vi "Create Request.vi"(8 "error in (no error)":errorcluster, 10 "request":T1, 11 "JSON-RPC in":refnum<class "JSON-RPC.lvclass">) -> (0 "error out":errorcluster, 2 "Request":string, 3 "JSON-RPC out":refnum<class "JSON-RPC.lvclass">)   [LabVIEW 2016, in "JSON-RPC.lvclass"]
uses:
  JSON-RPC.lvclass
  typedefs/Request--Cluster.ctl
  JSON-RPC.lvclass/JSON-RPC.ctl
  Request/Request.lvclass
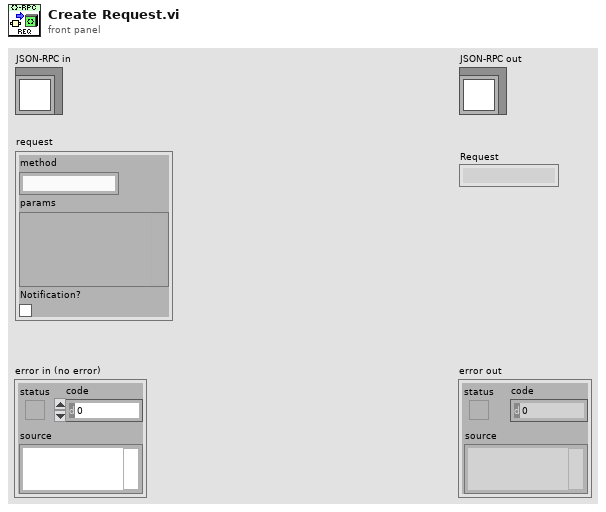
[diagram p1: front panel]
types:
  T1 = typedef "JSON-RPC.lvclass/Request--Cluster.ctl" = cluster{"method":string, "params":variant, "Notification?":bool}
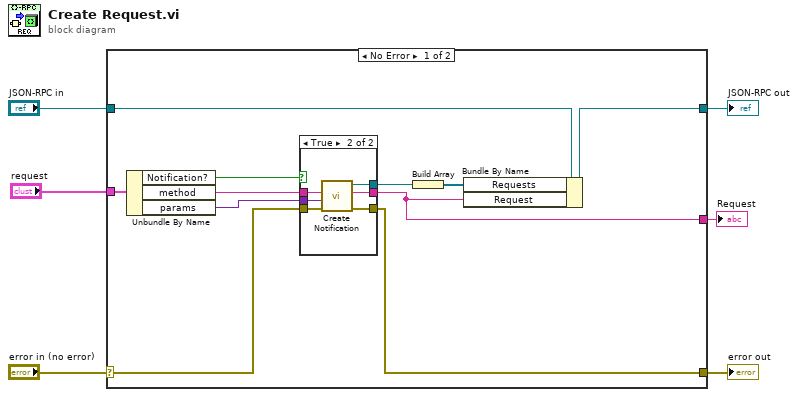
[diagram p0: block diagram]
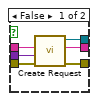
[diagram p2: hidden frame]
diagram:
  n1 = case shown="No Error" "error in (no error)" {
    selector: "error in (no error)" -> [w13 w31]
    tunnel: [w12 w31] -> w5
    tunnel: [w15 w30] -> w3
    tunnel: "JSON-RPC in" -> [w16 w30]
    tunnel: [w11 _] -> w2
    tunnel: "request" -> [w10 _]
    frame No Error {
      n2 = Unbundle By Name(w10) -> ("Notification?"=w9:bool, "method"=w7:string, "params"=w8:variant)
      n3 = case shown="True" w9 {
        tunnel: [w23 w27] -> w17
        tunnel: w8 -> [w22 w28]
        tunnel: w13 -> [w21 w29]
        tunnel: [w20 w25] -> w12
        tunnel: [w19 w26] -> w11
        tunnel: w7 -> [w18 w24]
        frame False {
          n4 = call "Create Request.vi"("error in (no error)"=w21, "params"=w22, "method"=w18) -> ("error out"=w20:errorcluster, "JSON Request"=w19:string, "Request out"=w23:refnum<class "Request.lvclass">)  [unwired: 6 in]
        }
        frame True {
          n5 = call "Create Notification.vi"("error in (no error)"=w29, "params"=w28, "method"=w24) -> ("error out"=w25:errorcluster, "JSON Notificaiton"=w26:string, "Request"=w27:refnum<class "Request.lvclass">)  [unwired: 6 in]
        }
      }
      n6 = Build Array(w17) -> (w14:refnum<class "Request.lvclass">[])
      n7 = Bundle By Name(cluster=w16, "Requests"=w14, "Request"=w11) -> (w15:refnum<class "JSON-RPC.lvclass">)
    }
    frame Error {
    }
  }
  "error out" <- w5
  "JSON-RPC out" <- w3
  "Request" <- w2
